vi "Parse PDR2000 Pressure String.vi"(11 "String":string) -> (2 "Pressure 2":dbl, 3 "Pressure 1":dbl)   [LabVIEW 2020, in "Gauge Control.lvclass"]
uses:
  Gauge Control.lvclass
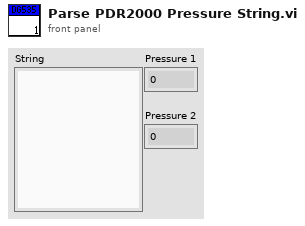
[diagram p1: front panel]
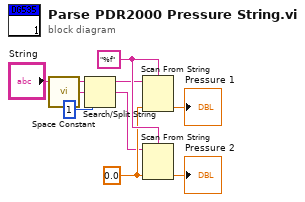
[diagram p0: block diagram]
diagram:
  w5 = 0.0 ("default value 2")
  w6 = "%f" ("format string")
  n1 = call "Space Constant.vi"() -> ("String"=w7:string)
  n2 = Search/Split String(string="String", search string/char (-)=w7, offset (0)=1) -> (substring before match=w3:string, match + rest of string=w4:string)  [unwired: 1 out]
  n3 = Scan From String(format string=w6, input string=w3, default 1=w5) -> (output 1=→"Pressure 1":dbl)  [unwired: 2 in, 3 out]
  n4 = Scan From String(format string=w6, input string=w4, default 1=w5) -> (output 1=→"Pressure 2":dbl)  [unwired: 2 in, 3 out]
